vi "Information.vi"(8 "error in (no error)":errorcluster, 9 "Context":T1, 10 "Information":refnum<class "Information.lvclass">, 11 "Communications in":refnum<class "Communications.lvclass">) -> (0 "error out":errorcluster, 3 "Communications out":refnum<class "Communications.lvclass">)   [LabVIEW 2021, in "Communications.lvclass"]
uses:
  Communications.lvclass
  Communications.lvclass/Communications.ctl
  NHMFL_Core/Libraries/Instruments/Results/Acquired Result/Acquired Result.lvclass
  Publish-Subscribe/Interfaces/Information/Information.lvclass
  Publish-Subscribe/Context.ctl
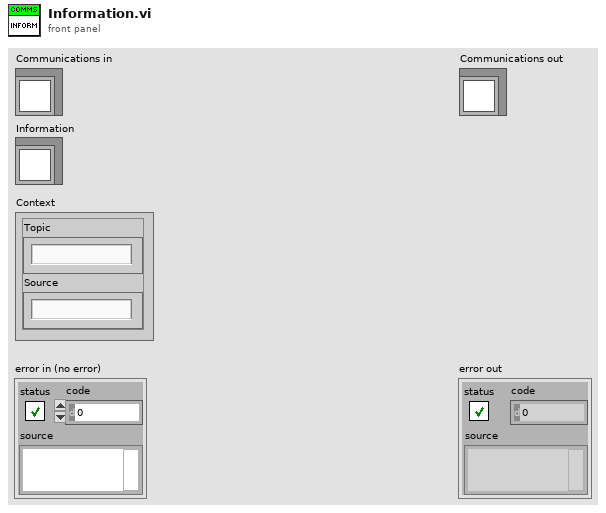
[diagram p1: front panel]
types:
  T1 = typedef "Context.ctl" = cluster{"Topic":string, "Source":string}
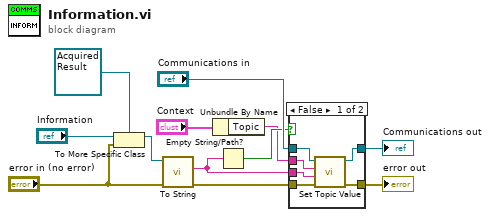
[diagram p0: block diagram]
diagram:
  n1 = To More Specific Class(target class=refnum<class "Acquired Result.lvclass"> refnum ("Acquired Result.lvclass"), reference="Information", error in="error in (no error)") -> (specific class reference=w3:refnum<class "Acquired Result.lvclass">)  [unwired: 1 out]
  n2 = call-dynamic "To String.vi"("error in (no error)"="error in (no error)", "Acquired Result in"=w3) -> ("error out"=w10:errorcluster, "String"=w8:string)  [unwired: 7 in, 1 out]
  n3 = Unbundle By Name("Context") -> ("Topic"=w1:string)
  n4 = Empty String/Path?(string/path=w8) -> (empty?=w7:bool)
  n5 = case shown="False" w7 {
    tunnel: "Communications in" -> [w18 w20]
    tunnel: [w17 w20] -> w11
    tunnel: w1 -> [w16 _]
    tunnel: w10 -> [w15 w19]
    tunnel: [w14 w19] -> w9
    tunnel: w8 -> [w13 _]
    frame False {
      n6 = call-dynamic "Set Topic Value.vi"("error in (no error)"=w15, "Value"=w13, "Topic"=w16, "Communications in"=w18) -> ("error out"=w14:errorcluster, "Communications out"=w17:refnum<class "Communications.lvclass">)  [unwired: 5 in, 1 out]
    }
    frame True {
    }
  }
  "error out" <- w9
  "Communications out" <- w11
